vi "settings_save_to_file.vi"(1 "Version":string, 10 "XML File Path":path) -> ()   [LabVIEW 2015]
uses:
  red_tweezers_globals_INTERNAL_VOLATILE.vi
  <vilib>/Utility/xml.llb/Write to XML File(array).vi
panel:
  out "VIs Saved":string[](array[string])
  out "error out":errorcluster
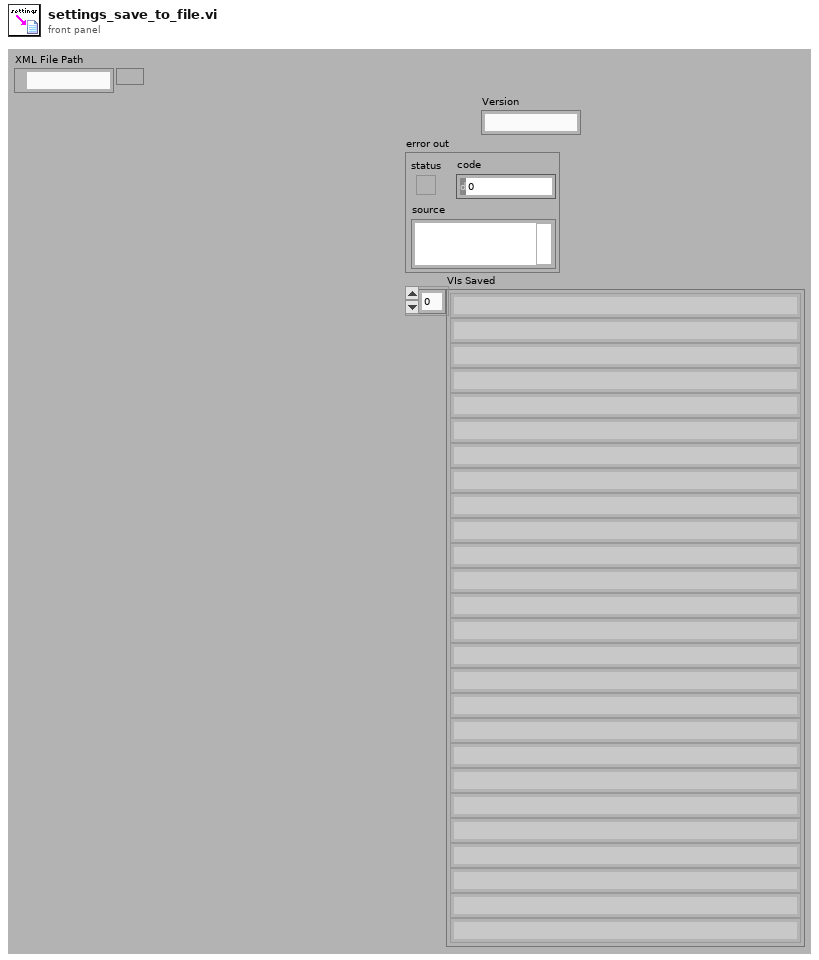
[diagram p1: front panel]
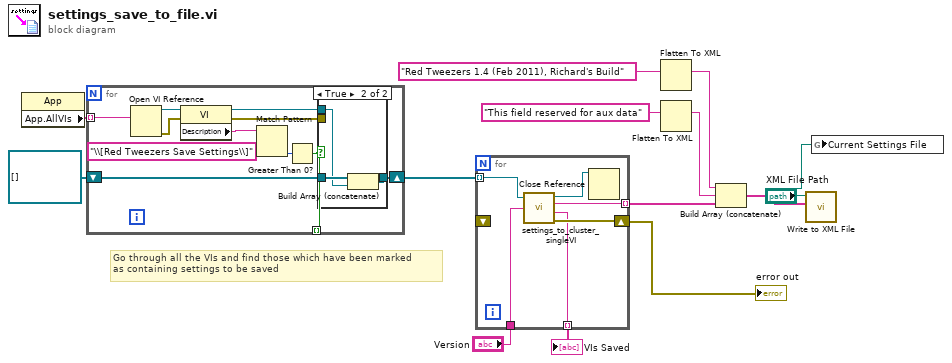
[diagram p0: block diagram]
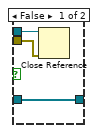
[diagram p2: hidden frame]
diagram:
  # "Go through all the VIs and find those which have been marked\nas containing settings to be saved"
  n1 = property class="App"() -> ("App.AllVIs"=w11:string[])  [unwired: 2 in, 2 out]
  n2 = for {
    tunnel: w11 -> [w22] mode=indexing
    shift-right: [w24] -> w9
    shift-left: refnum<vi>[] [] -> [w23]
    tunnel: [w15] -> _ mode=indexing
    n3 = Open VI Reference(vi path=w22) -> (vi reference=w21:refnum<vi>, error out=w20:errorcluster)  [unwired: 5 in]
    n4 = property class="VI"(reference=w21, error in=w20) -> (reference out=w17:refnum<vi>, error out=w16:errorcluster, "Description"=w14:string)
    n5 = Match Pattern(string=w14, regular expression="\\[Red Tweezers Save Settings\\]") -> (offset past match=w18:i32)  [unwired: 1 in, 3 out]
    n6 = Greater Than 0?(x=w18) -> (x > 0?=w15:bool)
    n7 = case shown="True" w15 {
      tunnel: [w25 w30] -> w24
      tunnel: w23 -> [w25 w29]
      tunnel: w17 -> [w27 w28]
      tunnel: w16 -> [w26 _]
      frame False {
        n8 = Close Reference(reference=w27, error in (no error)=w26) -> ()  [unwired: 1 out]
      }
      frame True {
        n9 = Build Array (concatenate)(w29, w28) -> (w30:refnum<vi>[])
      }
    }
  }
  n10 = for {
    tunnel: [w36] -> w13 mode=indexing
    shift-right: [w35] -> w12
    shift-left: _ -> [_]
    tunnel: w9 -> [w34] mode=indexing
    tunnel: "Version" -> [w33]
    tunnel: [w31] -> w6 mode=indexing
    n11 = call "settings_to_cluster_singleVI.vi"("Version"=w33, "vi reference 2"=w34) -> ("error out"=w35:errorcluster, "VI Name"=w31:string, "XML String"=w36:string, "vi reference"=w32:refnum<vi>)  [unwired: 1 in]
    n12 = Close Reference(reference=w32) -> ()  [unwired: 1 in, 1 out]
  }
  "error out" <- w12
  "VIs Saved" <- w6
  n13 = Flatten To XML(anything="Red Tweezers 1.4 (Feb 2011), Richard's Build" ("Version 2")) -> (xml string=w2:string)
  n14 = Flatten To XML(anything="This field reserved for aux data" ("Version 2")) -> (xml string=w3:string)
  n15 = Build Array (concatenate)(w2, w3, w13) -> (w7:string[])
  n16 = call-poly <vilib>:"Write to XML File.vi"("XML Input"=w7, "XML File Path"="XML File Path") -> ()  [unwired: 7 in, 3 out]
  n17 = global write "red_tweezers_globals_INTERNAL_VOLATILE.vi" "Current Settings File"("XML File Path") -> ()
